vi "Instrument.sendMessageToProcess (variant).vi"(6 "ID":string, 8 "error in (no error)":errorcluster, 9 "Data":variant, 10 "Command":variant, 11 "Instrument":refnum<class "Instrument.lvclass">) -> (0 "error out":errorcluster, 3 "Instrument out":refnum<class "Instrument.lvclass">)   [LabVIEW 2019, in "Instrument.lvlib" / "Instrument.lvclass"]
doc: "Send a message (<b>Command</b>, <b>Data</b>, <b>ID</b>) <b>to</b> Instrument.lvclass:process.vi\n\n<b>Command</b> should be a <b>string</b> or <b>enum</b>"
uses:
  Instrument.lvclass
  Typedefs/PrivateEvents--Instrument.MessageToProcess.ctl
  <userlib>/LevyLab/RemoteControl/Typedefs/Message--Cluster.ctl
  Instrument.lvclass/Instrument.ctl
  c3775509-5670-44bf-bc53-51ca81283145.vi
  <vilib>/Utility/Data Type/Get Type Information.vi
  <vilib>/Utility/Data Type/Get Numeric Information.vi
  <userlib>/_OpenG.lib/lvdata/lvdata.llb/Unwrap VVariant__ogtk.vi
  <userlib>/LevyLab/RemoteControl/RemoteControl.lvclass
panel:
  # "For instructions on how to use the JKI State Machine Objects, examples and video tutorials, visit:\nhttp://jki.net/state-machine-objects/\n\nJKI State Machine Objects™\nhttp://jki.net/state-machine-objects/\nCopyright (C) 2005-2015, JKI <info@jki.net>\nALL RIGHTS RESERVED"
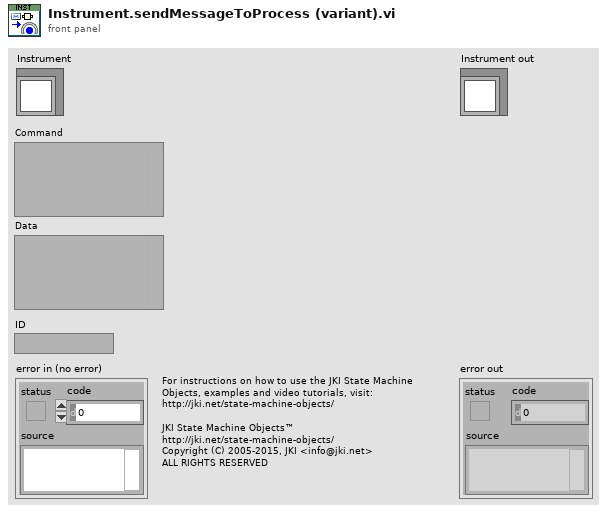
[diagram p1: front panel]
types:
  T1 = typedef "Instrument.lvlib/Instrument.lvclass/PrivateEvents--Instrument.MessageToProcess.ctl" = cluster{"Message":T2}
  T2 = typedef "RemoteControl.lvclass/Message--Cluster.ctl" = cluster{"Command":string, "Data":variant, "ID":string}
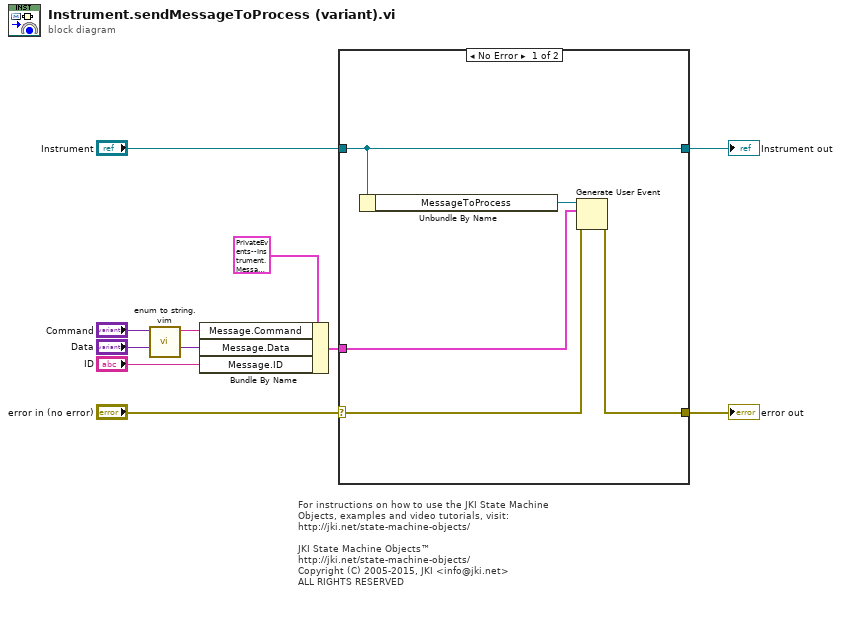
[diagram p0: block diagram]
diagram:
  # "For instructions on how to use the JKI State Machine Objects, examples and video tutorials, visit:\nhttp://jki.net/state-machine-objects/\n\nJKI State Machine Objects™\nhttp://jki.net/state-machine-objects/\nCopyright (C) 2005-2015, JKI <info@jki.net>\nALL RIGHTS RESERVED"
  n1 = call "enum to string.vim"("enum in"="Command") -> ("string out"=w2:string)  [unwired: 9 in, 1 out]
  n2 = Bundle By Name(cluster=T1 {"Message"={"Command"="", "Data"=variant(string ""), "ID"=""}} ("MessageToProcess"), "Message.Command"=w2, "Message.Data"="Data", "Message.ID"="ID") -> (w6:T1)
  n3 = case shown="No Error" "error in (no error)" {
    selector: "error in (no error)" -> [w15 w17]
    tunnel: [w13 w17] -> w9
    tunnel: [w12 w16] -> w10
    tunnel: "Instrument" -> [w12 w16]
    tunnel: w6 -> [w11 _]
    frame No Error {
      n4 = Unbundle By Name(w12) -> ("MessageToProcess"=w14:refnum<user-event>)
      n5 = Generate User Event(user event=w14, event data cluster=w11, error in=w15) -> (error out=w13:errorcluster)  [unwired: 1 in, 1 out]
    }
    frame Error {
    }
  }
  "error out" <- w9
  "Instrument out" <- w10
